vi "Verify JWT.vi"(8 "error in (no error)":errorcluster, 9 "Approved Algs":T1, 10 "Validate Times? (T)":bool=TRUE, 11 "Token":string) -> (0 "error out":errorcluster, 3 "Payload":string)   [LabVIEW 2020, in "JWT.lvlib" / "JWT.lvclass"]
uses:
  JWT.lvclass
  Algorithm Key Pairs.ctl
  Signature Algorithms.ctl
  lv-crypto/Crypto/Signature/Signature.lvclass
  JWT.lvlib
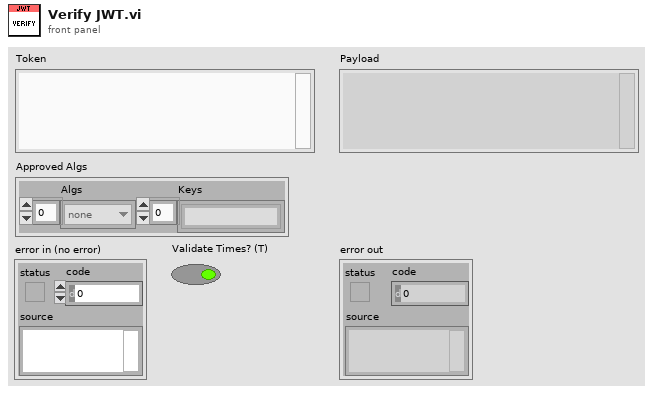
[diagram p1: front panel]
types:
  T1 = typedef "JWT.lvlib/Algorithm Key Pairs.ctl" = cluster{"Algs":T2[], "Keys":string[]}
  T2 = typedef "JWT.lvlib/Signature Algorithms.ctl" = enum16{"none", "HS256"}
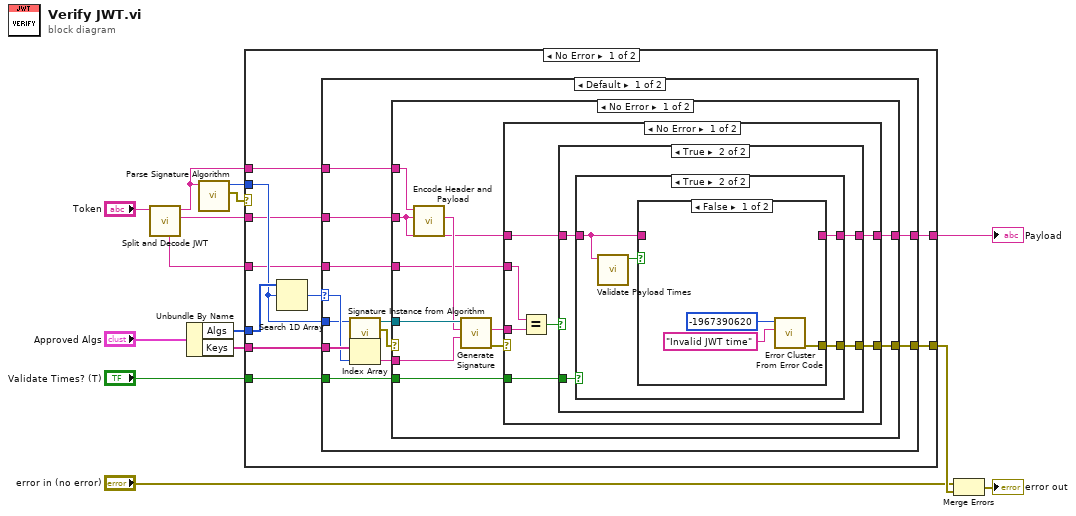
[diagram p0: block diagram]
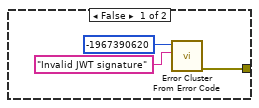
[diagram p2: hidden frame]
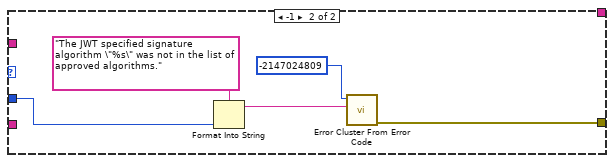
[diagram p7: hidden frame]
diagram:
  n1 = call "Split and Decode JWT.vi"("JWT"="Token") -> ("Payload JSON"=w2:string, "Header JSON"=w3:string, "Signature"=w1:string)  [unwired: 8 in]
  n2 = Unbundle By Name("Approved Algs") -> ("Algs"=w11:T2[], "Keys"=w10:string[])
  n3 = call "Parse Signature Algorithm.vi"("Header"=w3) -> ("error out"=w14:errorcluster, "Signature Algorithm"=w13:T2)  [unwired: 9 in]
  n4 = case shown="No Error" w14 {
    selector: w14 -> [_ w78]
    tunnel: w13 -> [w22 _]
    tunnel: w1 -> [w20 _]
    tunnel: w2 -> [w19 _]
    tunnel: w3 -> [w18 _]
    tunnel: w11 -> [w23 _]
    tunnel: w10 -> [w21 _]
    tunnel: [w17 w78] -> w9
    tunnel: [w16 _] -> w6
    tunnel: "Validate Times? (T)" -> [w15 _]
    frame No Error {
      n5 = Search 1D Array(1D array=w23, element=w22) -> (index of element=w24:i32)  [unwired: 1 in]
      n6 = case shown="Default" w24 {
        selector: w24 -> [w35 _]
        tunnel: w22 -> [w34 w75]
        tunnel: [w31 w73] -> w17
        tunnel: w21 -> [w36 _]
        tunnel: w20 -> [w29 _]
        tunnel: w19 -> [w28 _]
        tunnel: w18 -> [w27 _]
        tunnel: [w26 _] -> w16
        tunnel: w15 -> [w25 _]
        frame Default {
          n7 = call "Signature Instance from Algorithm.vi"("Signature Algorithm"=w34) -> ("error out"=w32:errorcluster, "Signature"=w33:refnum<class "Signature.lvclass">)  [unwired: 9 in]
          n8 = Index Array(array=w36, index=w35) -> (element=w30:string)
          n9 = case shown="No Error" w32 {
            selector: w32 -> [_ w72]
            tunnel: w33 -> [w47 _]
            tunnel: [w39 w72] -> w31
            tunnel: w30 -> [w46 _]
            tunnel: w29 -> [w41 _]
            tunnel: w28 -> [w40 _]
            tunnel: w27 -> [w44 _]
            tunnel: [w38 _] -> w26
            tunnel: w25 -> [w37 _]
            frame No Error {
              n10 = call "Encode Header and Payload.vi"("Payload"=w40, "Header"=w44) -> ("Encoded"=w45:string)  [unwired: 9 in]
              n11 = call-dynamic "Generate Signature.vi"("Key"=w46, "Message"=w45, "Signature in"=w47) -> ("error out"=w43:errorcluster, "Signature"=w42:string)  [unwired: 6 in, 1 out]
              n12 = case shown="No Error" w43 {
                selector: w43 -> [_ w71]
                tunnel: w42 -> [w54 _]
                tunnel: w41 -> [w53 _]
                tunnel: w40 -> [w52 _]
                tunnel: [w49 w71] -> w39
                tunnel: [w50 _] -> w38
                tunnel: w37 -> [w48 _]
                frame No Error {
                  n13 = Equal?(x=w53, y=w54) -> (x = y?=w51:bool)
                  n14 = case shown="True" w51 {
                    tunnel: w52 -> [_ w60]
                    tunnel: [_ w59] -> w50
                    tunnel: [w57 w58] -> w49
                    tunnel: w48 -> [_ w61]
                    frame False {
                      n15 = call <vilib>:"Error Cluster From Error Code.vi"("error message (\"\")"="Invalid JWT signature", "error code (0)"=-1967390620) -> ("error out"=w57:errorcluster)  [unwired: 7 in]
                    }
                    frame True {
                      n16 = case shown="True" w61 {
                        tunnel: w60 -> [w62 w66]
                        tunnel: [w62 w64] -> w59
                        tunnel: [_ w63] -> w58
                        frame False {
                        }
                        frame True {
                          n17 = call "Validate Payload Times.vi"("Payload"=w66) -> ("Times Valid"=w65:bool)  [unwired: 10 in]
                          n18 = case shown="False" w65 {
                            tunnel: w66 -> [_ w70]
                            tunnel: [_ w70] -> w64
                            tunnel: [w67 _] -> w63
                            frame False {
                              n19 = call <vilib>:"Error Cluster From Error Code.vi"("error message (\"\")"="Invalid JWT time", "error code (0)"=-1967390620) -> ("error out"=w67:errorcluster)  [unwired: 7 in]
                            }
                            frame True {
                            }
                          }
                        }
                      }
                    }
                  }
                }
                frame Error {
                }
              }
            }
            frame Error {
            }
          }
        }
        frame -1 {
          n20 = Format Into String(format string="The JWT specified signature algorithm \"%s\" was not in the list of approved algorithms.", w75) -> (resulting string=w74:string)  [unwired: 2 in, 1 out]
          n21 = call <vilib>:"Error Cluster From Error Code.vi"("error message (\"\")"=w74, "error code (0)"=-2147024809) -> ("error out"=w73:errorcluster)  [unwired: 7 in]
        }
      }
    }
    frame Error {
    }
  }
  "Payload" <- w6
  n22 = Merge Errors("error in (no error)", w9) -> (→"error out":errorcluster)
